vi "GL_DRCtype.vi"() -> ()   [LabVIEW 2019]
panel:
  in  "CONTROLLER TYPE":bool
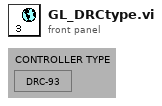
[diagram p1: front panel]
diagram:
